vi "FSET.vi"(8 "error in (no error)":errorcluster, 10 "Function (0: Cp-D)":u16(ring) items=["Cp-D", "Cp-Q", "Cp-G", "Cp-Rp", "Cs-D", "Cs-Q", "Cs-Rs", "Lp-D", "Lp-Q", "Lp-G", "Lp-Rp", "Lp-Rdc", "Ls-D", "Ls-Q", "Ls-Rs", "Ls-Rdc", "R-X", "Z-thd", "Z-thr", "G-B", "Y-thd", "Y-thr", "Vdc-Idc"], 11 "VISA resource name":refnum<visa-resource-name>) -> (0 "error out":errorcluster, 3 "VISA resource name out":refnum<visa-resource-name>)   [LabVIEW 2017]
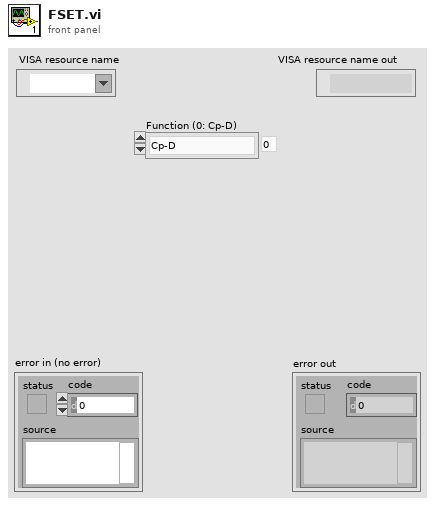
[diagram p1: front panel]
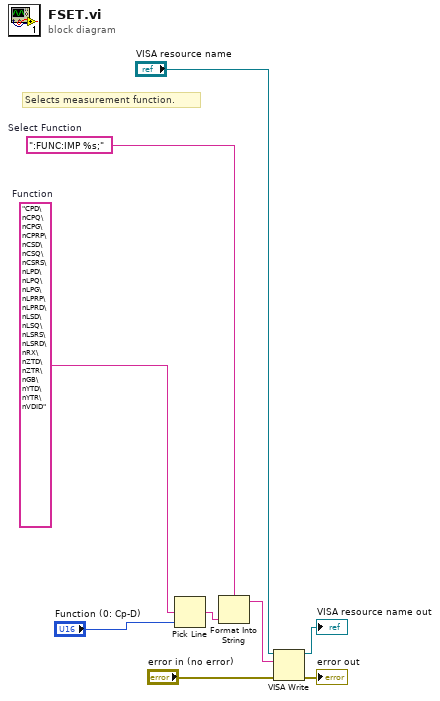
[diagram p0: block diagram]
diagram:
  w5 = ":FUNC:IMP %s;"  # Select Function
  w7 = "CPD\nCPQ\nCPG\nCPRP\nCSD\nCSQ\nCSRS\nLPD\nLPQ\nLPG\nLPRP\nLPRD\nLSD\nLSQ\nLSRS\nLSRD\nRX\nZTD\nZTR\nGB\nYTD\nYTR\nVDID"  # Function
  # "Selects measurement function."
  n1 = Pick Line(multi-line string=w7, line index="Function (0: Cp-D)") -> (output string=w4:string)  [unwired: 1 in]
  n2 = Format Into String(format string=w5, w4) -> (resulting string=w3:string)  [unwired: 2 in, 1 out]
  n3 = VISA Write(VISA resource name="VISA resource name", write buffer=w3, error in (no error)="error in (no error)") -> (VISA resource name out=→"VISA resource name out":refnum<visa-resource-name>, error out=→"error out":errorcluster)  [unwired: 1 out]
